vi "Control Transfer Release.vi"(11 "Avoid Race Condition":bool) -> ()   [LabVIEW 2020]
uses:
  Framework/Robot Global Data.vi
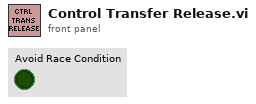
[diagram p1: front panel]
types:
  T1 = typedef "Command Status Info.ctl" = cluster{"Name":string, "Status":T2, "notifier out":T3}
  T2 = typedef "Completion Status.ctl" = enum16{"Successful", "Aborted", "Incomplete"}
  T3 = typedef "Completion Notifier.ctl" = refnum<notifier>
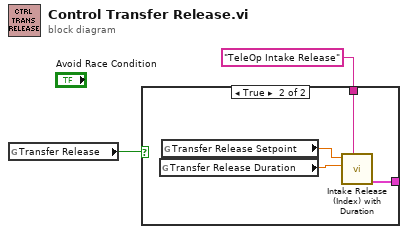
[diagram p0: block diagram]
diagram:
  n1 = global read "Robot Global Data.vi" "Transfer Release"() -> (w1:bool)
  n2 = case shown="True" w1 {
    tunnel: [_ w4] -> _
    tunnel: "TeleOp Intake Release" ("Description") -> [_ w3]
    frame False {
    }
    frame True {
      n3 = global read "Robot Global Data.vi" "Transfer Release Duration"() -> (w5:dbl)
      n4 = global read "Robot Global Data.vi" "Transfer Release Setpoint"() -> (w6:dbl)
      n5 = call "Intake Release (Index) with Duration.vi"("Description"=w3, "Duration (s)"=w5, "Setpoint"=w6) -> ("Command Info Out"=w4:T1)  [unwired: 8 in]
    }
  }
